vi "get update log.vi"(8 "error in (no error)":errorcluster caption="错误输入（无错误）", 11 "服务器信息":T1={"host"="27.154.58.30", "user"="fb", "password"="std23506", "远端地址"="/微站/室外总磷总氮高压过滤无主板新电路板/一体化微型水质监测站.exe"}) -> (0 "error out":errorcluster caption="错误输出", 1 "部分更新日志":string, 2 "remote File Version":string, 3 "更新日志":string)   [LabVIEW 2016, in "update.lvlib"]
uses:
  update.lvlib
  <vilib>/regexp/Match Regular Expression.xnode
  <vilib>/FTP/NI_FTP.lvlib
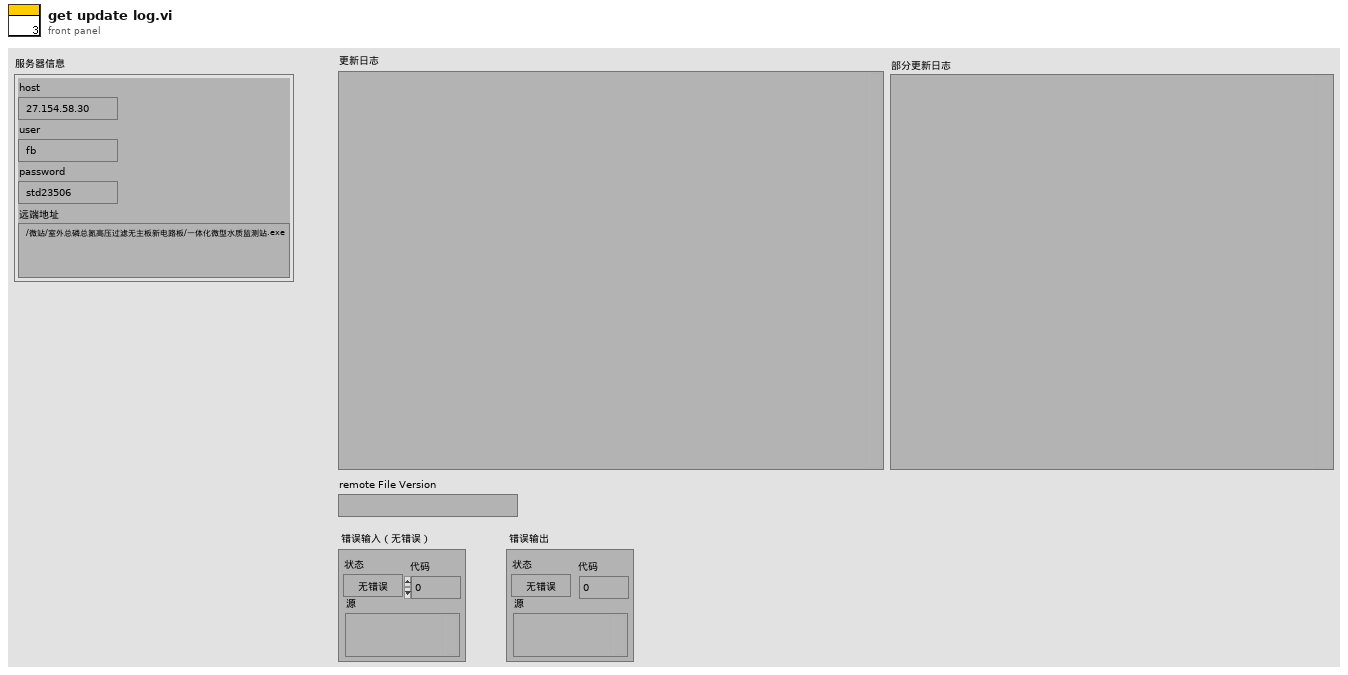
[diagram p1: front panel]
types:
  T1 = cluster{"host":string, "user":string, "password":string, "远端地址":string}
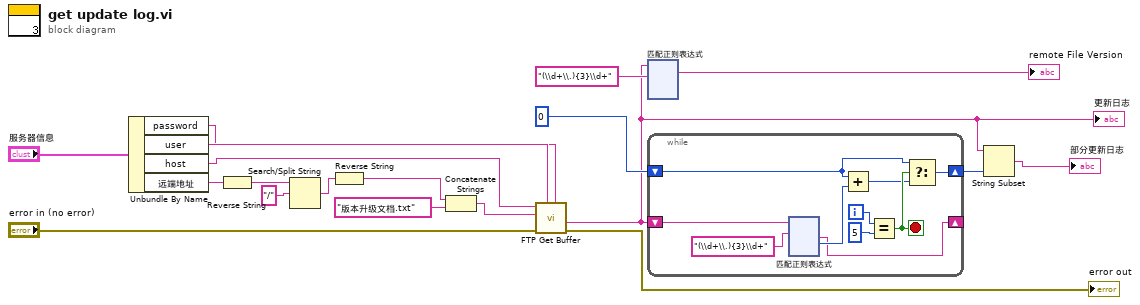
[diagram p0: block diagram]
diagram:
  n1 = Unbundle By Name("服务器信息") -> ("password"=w16:string, "user"=w17:string, "host"=w15:string, "远端地址"=w11:string)
  n2 = Reverse String(1:w11) -> (0:w10:string)
  n3 = Search/Split String(string=w10, search string/char (-)="/" ("搜索字符串/字符(-)")) -> (match + rest of string=w8:string)  [unwired: 1 in, 2 out]
  n4 = Reverse String(1:w8) -> (0:w7:string)
  n5 = Concatenate Strings(w7, "版本升级文档.txt" ("字符串")) -> (w5:string)
  n6 = call <vilib>:"FTP Get Buffer.vi"("password"=w16, "user"=w17, "error in (no error)"="error in (no error)", "remote path"=w5, "host"=w15) -> ("error out"=→"error out":errorcluster, "data"=w3:string)  [unwired: 4 in, 1 out]
  "更新日志" <- w3
  n7 = xnode "匹配正则表达式"("输入字符串"=w3, "正则表达式"="(\\d+\\.){3}\\d+") -> ("所有匹配"=→"remote File Version":string)  [unwired: 4 in, 4 out]
  n8 = while {
    shift-right: [w23] -> _
    shift-left: w3 -> [w28]
    shift-right: [w24] -> w2
    shift-left: 0 ("匹配后偏移量") -> [w21]
    i -> [w20]
    stop <- w26 stop-if-true
    n9 = xnode "匹配正则表达式"("输入字符串"=w28, "正则表达式"="(\\d+\\.){3}\\d+") -> ("匹配之后"=w23:string, "匹配后偏移量"=w25:i32)  [unwired: 4 in, 3 out]
    n10 = Add(x=w21, y=w25) -> (x+y=w22:i32)
    n11 = Equal?(x=w20, y=5) -> (x = y?=w26:bool)
    n12 = Select(t=w21, s=w26, f=w22) -> (s? t:f=w24:i32)
  }
  n13 = String Subset(string=w3, length (rest)=w2) -> (substring=→"部分更新日志":string)  [unwired: 1 in]
